vi "set state.vi"(8 "error in (no error)":errorcluster, 11 "new_state":u32(ring) items=["UNINITIALIZED", "RUNNING", "PAUSED", "EXITING"]) -> (0 "error out":errorcluster, 3 "function return":i32)   [LabVIEW 2014, in "test_IMU.lvlib"]
doc: "int set_state(state_t new_state);"
uses:
  <userlib>/test_IMU/test_IMU.lvlib
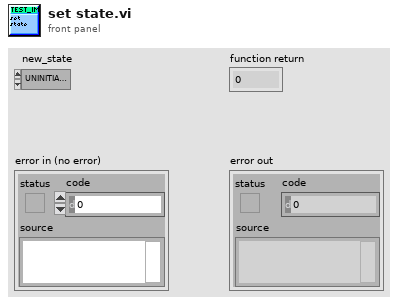
[diagram p1: front panel]
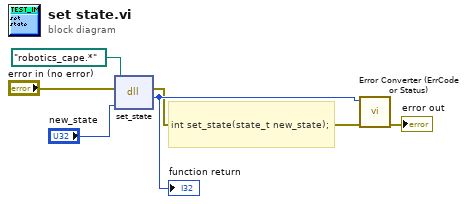
[diagram p0: block diagram]
diagram:
  # "int set_state(state_t new_state);"
  n1 = dll-call lib="C:/Users/ktalke/Documents/Updated Header File/6.18.16/Compiled SO -schroot/robotics_cape.so" fn="set_state"(path in=path "robotics_cape.*", error in="error in (no error)", "new_state"="new_state") -> (error out=w3:errorcluster, "return type"=w6:i32)  [unwired: 2 in, 1 out]
  "function return" <- w6
  n2 = call <userlib>:"Error Converter (ErrCode or Status).vi"("error in (no error)"=w3, "error code"=w6) -> ("error out"=→"error out":errorcluster)  [unwired: 9 in]
